vi "Main.vi"(10 "DAQ Type":enum16{"Hardware", "Simulation"}(ring), 11 "Module Admin":refnum<class "Delacor_lib_QMH_Module Admin.lvclass">) -> ()   [LabVIEW 2016, in "DAQ Hardware.lvlib"]
doc: "This template is based off of the Queued Message Handler design pattern and the Queued Message Handler project template that ships with LabVIEW.\n\nThe main difference is that the queue is private to this module and communication between modules is performed via Broadcast and Request events.\n\nRequest events are wrapped in public API methods and are handled in the Event Handling Loop (EHL) of this VI. Any module can register for Broadcast events sent by this module. The EHL generates messages based on user interface actions.\n\nThe Message Handling Loop (MHL) processes messages generated by the EHL, or by other messages. The messages are string values, so new messages can be added easily to the Message Cases case structure in the MHL. Each message cluster can also provide an optional value for Message Data, which is a variant that can be converted to whatever message-specific data is required.\n_____\nBased on DQMH Project Template 6.1.0.94."
uses:
  DAQ Hardware.lvlib
  <vilib>/Delacor/Delacor QMH/Libraries/Module Admin_class/Delacor_lib_QMH_Module Admin.lvclass
  Class/PXIe 6363/PXIe 6363.lvclass
  D:/common_ATE/Libraries/DAQ Hardware/Class/Abstract/Abstract.lvclass
  Module Data--cluster.ctl
  Class/Abstract/Abstract.lvclass
  User Interface/AI Channel Setting.ctl
  Timing AI DAQ Setting.ctl
  DI Channel Setting.ctl
  DO Channel Setting.ctl
  AO Channel Setting.ctl
  <vilib>/Delacor/Delacor QMH/Libraries/Message Queue_class/Delacor_lib_QMH_Message Queue.lvclass/Delacor_lib_QMH_Message Queue.ctl
  Stop Argument--cluster.ctl
  <vilib>/Delacor/Delacor QMH/Libraries/Module Admin_class/Delacor_lib_QMH_Module Admin.lvclass/Delacor_lib_QMH_Module Admin.ctl
  REQ Initialize AI Argument--cluster.ctl
  REQ Initialize AI (Reply Payload)--cluster.ctl
  REQ Initialize AO Argument--cluster.ctl
  REQ Initialize AO (Reply Payload)--cluster.ctl
  REQ Initialize DI Argument--cluster.ctl
  REQ Initialize DI (Reply Payload)--cluster.ctl
  REQ Initialize DO Argument--cluster.ctl
  REQ Initialize DO (Reply Payload)--cluster.ctl
  REQ Write DO Argument--cluster.ctl
  REQ Acquire AI Argument--cluster.ctl
  REQ Close Ref Argument--cluster.ctl
  REQ Write AO Argument--cluster.ctl
  REQ Update Sample Rate Argument--cluster.ctl
  REQ Acquire DI Argument--cluster.ctl
  <vilib>/Utility/miscctls.llb/LVPointTypeDef.ctl
  <vilib>/Delacor/Delacor QMH/Libraries/Message Queue_class/Delacor_lib_QMH_Enqueue Message (Single).vi
  <vilib>/Delacor/Delacor QMH/Libraries/Module Admin_class/Delacor_lib_QMH_Get External Launch.vi
  Support Global.vi
  <vilib>/Utility/error.llb/Error Cluster From Error Code.vi
  <vilib>/ErrorRing/Error Ring.xnode
  <vilib>/Delacor/Delacor QMH/Libraries/Message Queue_class/Delacor_lib_QMH_Message Queue.lvclass
  User Interface/User Interface.lvlib
panel:
  in  "Acquire DI":bool
  out "AI Data":dbl[][](graph)
  in  "Acquire AI":bool
  out "error out":errorcluster
  out "Status":string
  in  "Simulate MHL Error":bool
  in  "Simulate EHL Error":bool
  # "Other QMH Modules communicate with this Module via its Public API (wrappers for its Request Events).\n\nThis Module communicates with other Modules via its Broadcast Events.\nAny module that wants to get these messages, just registers for this module's Broadcast events."
  # "This template is for the Delacor Modified Queued Message Handler design pattern.\n\nSee the block diagram for more information on how to use this template."
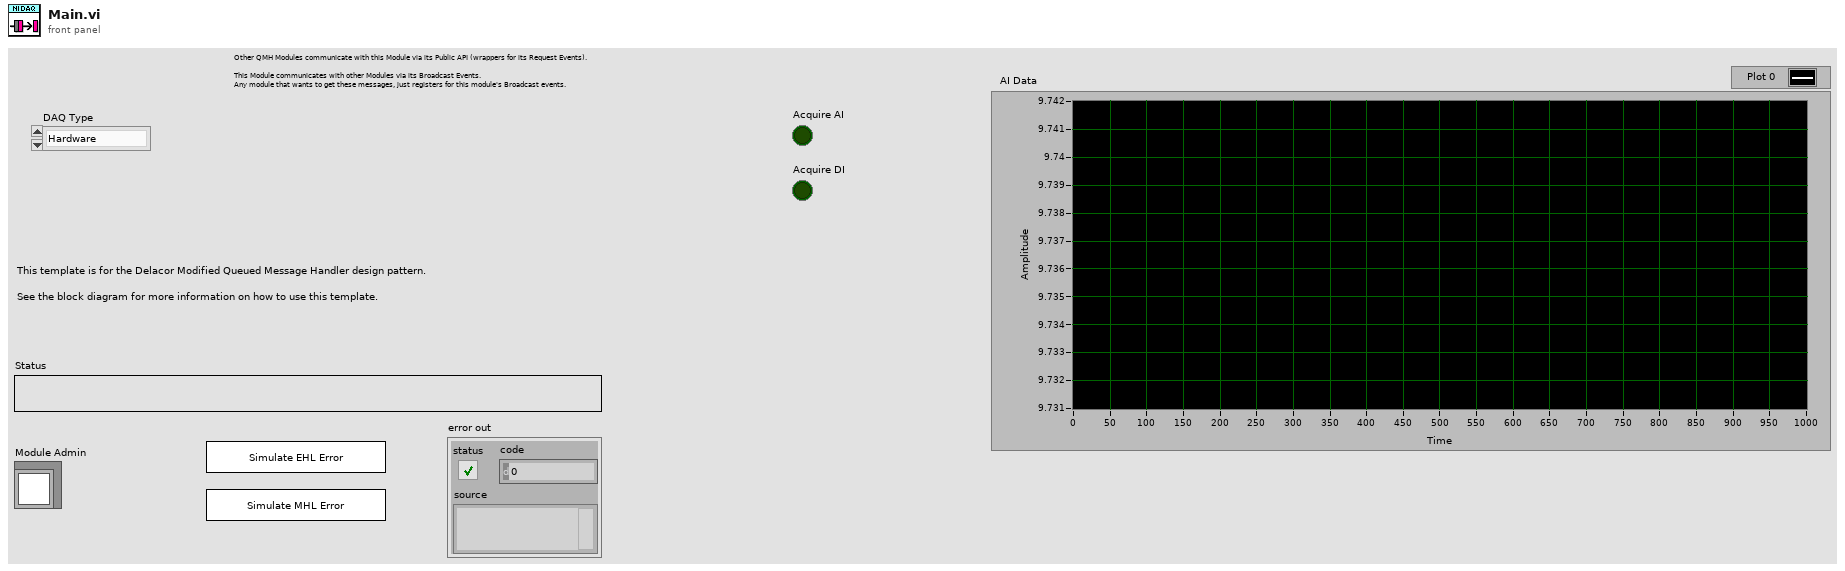
[diagram p1: front panel]
types:
  T1 = typedef "DAQ Hardware.lvlib/Module Data--cluster.ctl" = cluster{"Status":string, "Abstract.lvclass":refnum<class "Abstract.lvclass">, "AI Setting":T2, "Timing Parameter":T3, "DI Channel Setting":T4, "DO Channel Setting":T5, "AO Channel Setting":T6}
  T2 = typedef "DAQ Hardware.lvlib/AI Channel Setting.ctl" = cluster{"Physical Channel":string[], "Name to assign":string[], "input terminal configuration":enum16{"RSE", "NRSE", "Differential"}, "minimum value":dbl, "maximum value":dbl, "units":enum16{"Volts"}, "custom scale name":string, "sample mode":enum16{"Finite Samples", "Continuous Samples", "Hardware Timed Single Point"}, "rate":dbl, "samples per channel":dbl}
  T3 = typedef "DAQ Hardware.lvlib/Timing AI DAQ Setting.ctl" = cluster{"rate":dbl, "samples per channel":i32, "sample mode":i32}
  T4 = typedef "DAQ Hardware.lvlib/DI Channel Setting.ctl" = cluster{"DI Channel":string[]}
  T5 = typedef "DAQ Hardware.lvlib/DO Channel Setting.ctl" = cluster{"DO Channel":string[]}
  T6 = typedef "DAQ Hardware.lvlib/AO Channel Setting.ctl" = cluster{"AO Channel name":string[], "output terminal configuration":enum16{"RSE", "NRSE", "Differential"}, "minimum value":dbl, "maximum value":dbl, "units":enum16{"Volts"}, "name to assign":string[]}
  T7 = typedef "DAQ Hardware.lvlib/Request Events--cluster.ctl" = cluster{"Stop Module":refnum<user-event>, "Show Panel":refnum<user-event>, "Hide Panel":refnum<user-event>, "Get Module Execution Status":refnum<user-event>, "Show Diagram":refnum<user-event>, "REQ Initialize AI":refnum<user-event>, "REQ Initialize AO":refnum<user-event>, "REQ Initialize DI":refnum<user-event>, "REQ Initialize DO":refnum<user-event>, "REQ Write DO":refnum<user-event>, "REQ Acquire AI":refnum<user-event>, "REQ Close Ref":refnum<user-event>, "REQ Write AO":refnum<user-event>, "REQ Update Sample Rate":refnum<user-event>, "REQ Acquire DI":refnum<user-event>}
  T8 = enum32{"invalid lock state", "Not Locked", "Locked (No Password)", "Password-protected"}
  T9 = typedef "DAQ Hardware.lvlib/Stop Argument--cluster.ctl" = cluster{"Origin":string, "Exit via Stop Module Req?":bool, "Wait for Module to stop?":bool}
  T10 = typedef "DAQ Hardware.lvlib/REQ Initialize AI Argument--cluster.ctl" = cluster{"Wait Notifier":refnum<notifier>, "wait for reply":bool, "AI Setting":T2}
  T11 = typedef "DAQ Hardware.lvlib/REQ Initialize AO Argument--cluster.ctl" = cluster{"Boolean":bool, "Wait Notifier":refnum<notifier>, "wait for reply":bool, "AO Channel Setting":T6}
  T12 = typedef "DAQ Hardware.lvlib/REQ Initialize DI Argument--cluster.ctl" = cluster{"Boolean":bool, "Wait Notifier":refnum<notifier>, "wait for reply":bool, "DI Channel Setting":T4}
  T13 = typedef "DAQ Hardware.lvlib/REQ Initialize DO Argument--cluster.ctl" = cluster{"Boolean":bool, "Wait Notifier":refnum<notifier>, "wait for reply":bool, "DO Channel Setting":T5}
  T14 = typedef "DAQ Hardware.lvlib/REQ Write DO Argument--cluster.ctl" = cluster{"DO Value":bool[]}
  T15 = typedef "DAQ Hardware.lvlib/REQ Acquire AI Argument--cluster.ctl" = cluster{"Acquire AI":bool}
  T16 = typedef "DAQ Hardware.lvlib/REQ Close Ref Argument--cluster.ctl" = cluster{"Boolean":bool}
  T17 = typedef "DAQ Hardware.lvlib/REQ Write AO Argument--cluster.ctl" = cluster{"Value":dbl[]}
  T18 = typedef "DAQ Hardware.lvlib/REQ Update Sample Rate Argument--cluster.ctl" = cluster{"Timing Parameter":T3}
  T19 = typedef "DAQ Hardware.lvlib/REQ Acquire DI Argument--cluster.ctl" = cluster{"Acquire DI":bool}
  T20 = typedef "LVPointTypeDef.ctl" = cluster{"Horizontal":i16, "Vertical":i16}
  T21 = enum32{"Invalid", "Standard", "Closed", "Hidden", "Minimized", "Maximized"}
  T22 = typedef "DAQ Hardware.lvlib/REQ Initialize AI (Reply Payload)--cluster.ctl" = cluster{"error":errorcluster, "Connect?":bool}
  T23 = typedef "DAQ Hardware.lvlib/REQ Initialize AO (Reply Payload)--cluster.ctl" = cluster{"error":errorcluster, "Connect?":bool}
  T24 = typedef "DAQ Hardware.lvlib/REQ Initialize DI (Reply Payload)--cluster.ctl" = cluster{"error":errorcluster, "Connect?":bool}
  T25 = typedef "DAQ Hardware.lvlib/REQ Initialize DO (Reply Payload)--cluster.ctl" = cluster{"error":errorcluster, "Connect?":bool}
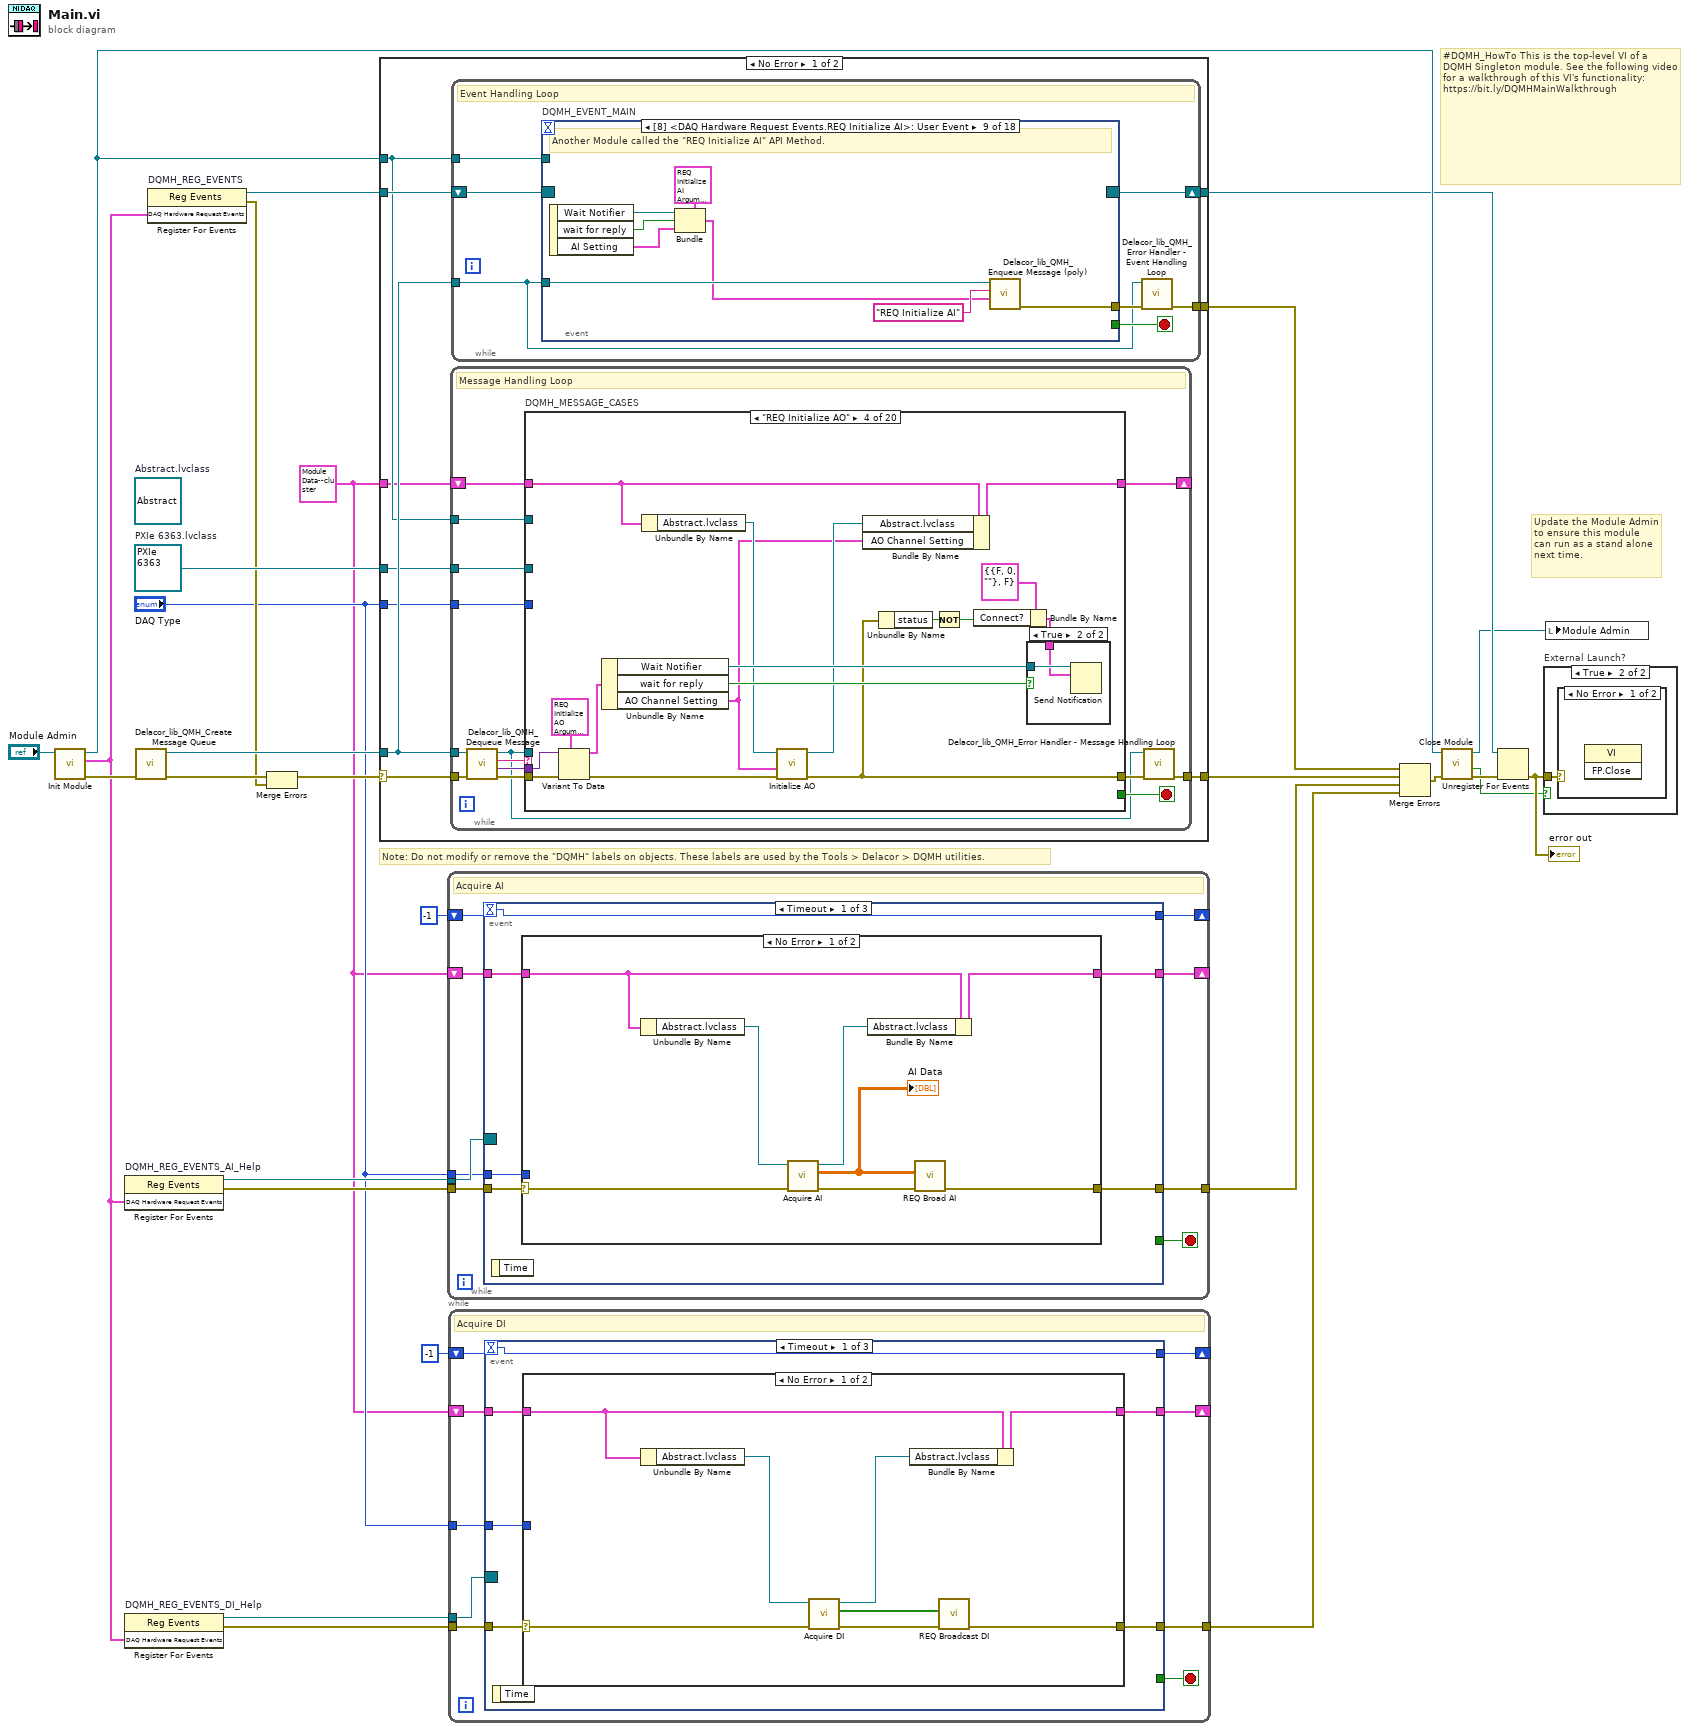
[diagram p0: block diagram]
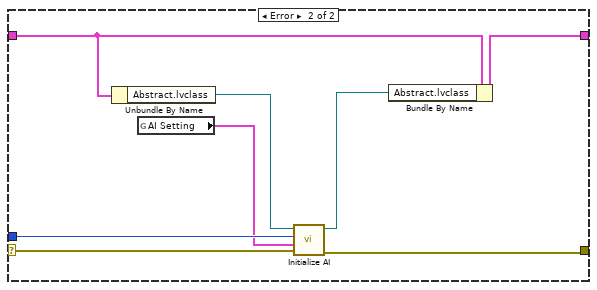
[diagram p2: hidden frame]
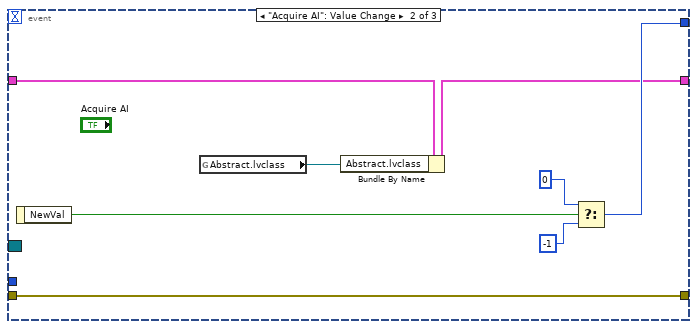
[diagram p3: hidden frame]
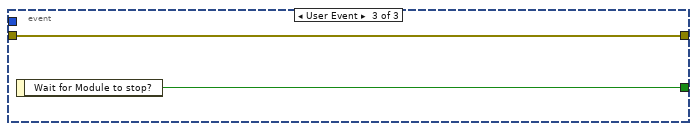
[diagram p4: hidden frame]
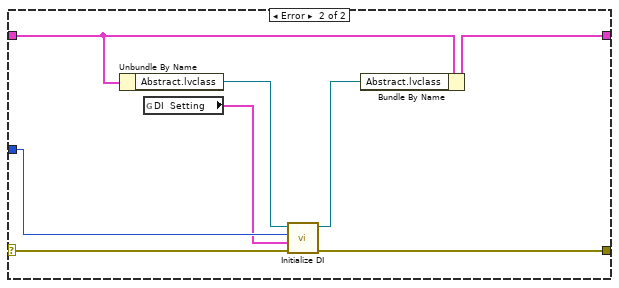
[diagram p5: hidden frame]
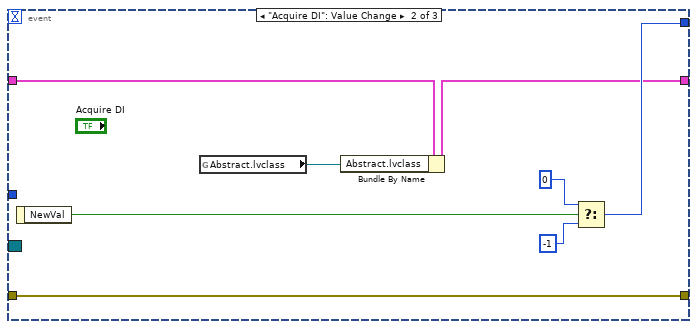
[diagram p6: hidden frame]
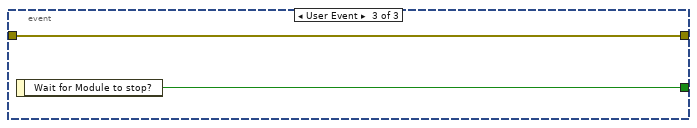
[diagram p7: hidden frame]
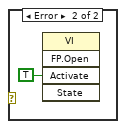
[diagram p9: hidden frame]
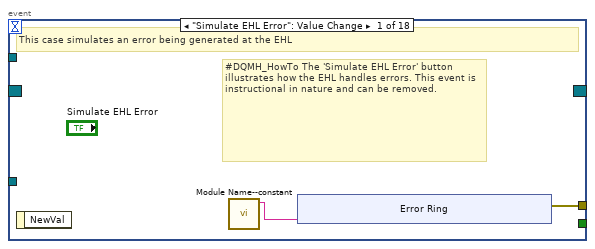
[diagram p10: hidden frame]
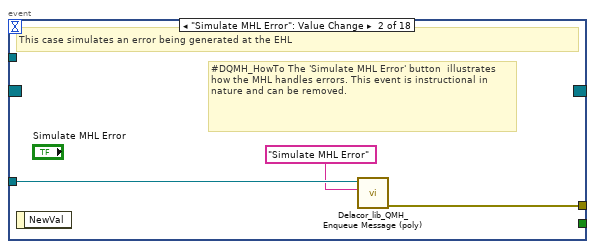
[diagram p11: hidden frame]
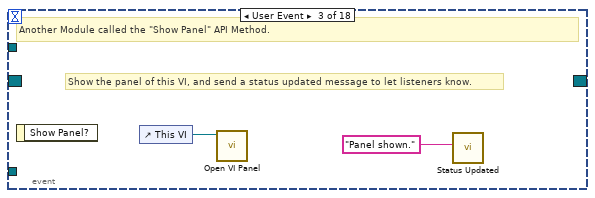
[diagram p12: hidden frame]
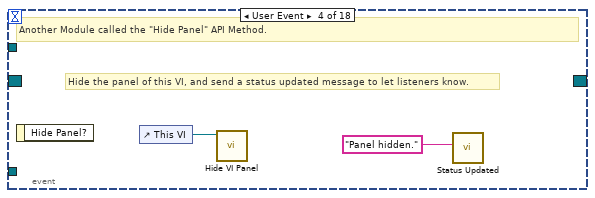
[diagram p13: hidden frame]
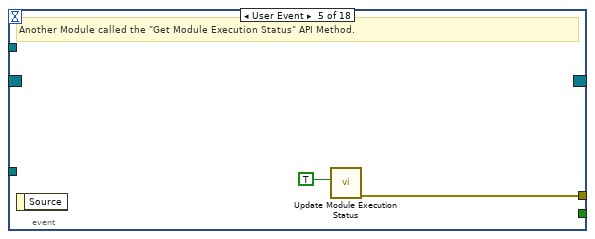
[diagram p14: hidden frame]
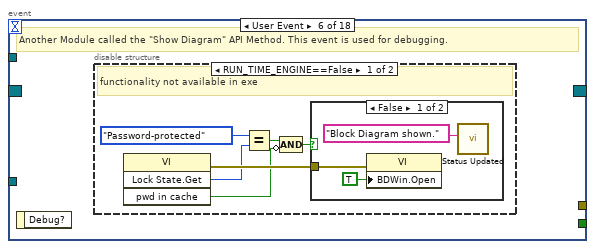
[diagram p15: hidden frame]
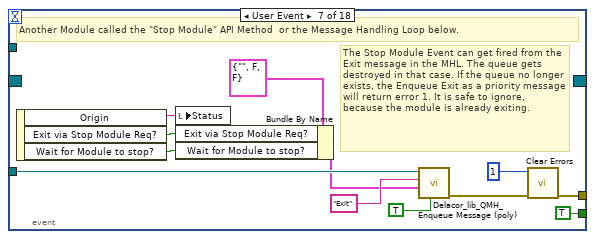
[diagram p18: hidden frame]
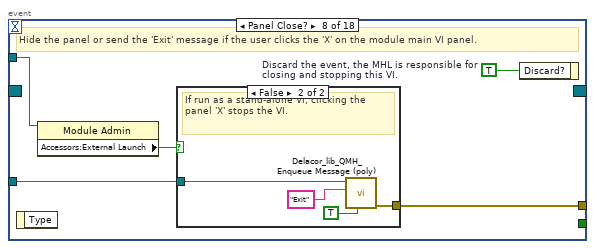
[diagram p19: hidden frame]
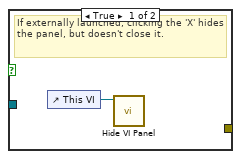
[diagram p20: hidden frame]
diagram:
  w1 = T1 {"Status"="", "Abstract.lvclass"=refnum, "AI Setting"={"Physical Channel"=["6363/ai0", "6363/ai1", "6363/ai2"], "Name to assign"=[], "input terminal configuration"=enum."RSE", "minimum value"=0.0, "maximum value"=10.0, "units"=enum."Volts", "custom scale name"="", "sample mode"=enum."Finite Samples", "rate"=5000.0, "samples per channel"=1000.0}, "Timing Parameter"={"rate"=1000.0, "samples per channel"=1000, "sample mode"=10123}, "DI Channel Setting"={"DI Channel"=[]}, "DO Channel Setting"={"DO Channel"=[]}, "AO Channel Setting"={"AO Channel name"=[], "output terminal configuration"=enum."RSE", "minimum value"=-10.0, "maximum value"=10.0, "units"=enum."Volts", "name to assign"=[]}} ("Data Cluster")
  w18 = refnum<class "PXIe 6363.lvclass"> refnum  # PXIe 6363.lvclass
  (unwired) refnum<class "Abstract.lvclass"> refnum  # Abstract.lvclass
  # "#DQMH_HowTo This is the top-level VI of a DQMH Singleton module. See the following video for a walkthrough of this VI's functionality: https://bit.ly/DQMHMainWalkthrough"
  # "Note: Do not modify or remove the \"DQMH\" labels on objects. These labels are used by the Tools > Delacor > DQMH utilities."
  # "Update the Module Admin to ensure this module can run as a stand alone next time."
  n1 = call "Init Module.vi"("Singleton Module Admin in"="Module Admin") -> ("error out"=w15:errorcluster, "DAQ Hardware Request Events"=w6:T7, "Singleton Module Admin out"=w23:refnum<class "Delacor_lib_QMH_Module Admin.lvclass">)  [unwired: 8 in]
  n2 = register-events "DQMH_REG_EVENTS_AI_Help"(w6) -> (reference out=w11:refnum<event-registration>, error out=w10:errorcluster)  [unwired: 2 in]
  n3 = register-events "DQMH_REG_EVENTS_DI_Help"(w6) -> (reference out=w5:refnum<event-registration>, error out=w4:errorcluster)  [unwired: 2 in]
  n4 = call <vilib>:"Delacor_lib_QMH_Create Message Queue.vi"("error in"=w15) -> ("error out"=w16:errorcluster, "Message Queue"=w17:refnum<class "Delacor_lib_QMH_Message Queue.lvclass">)  [unwired: 9 in]
  n5 = register-events "DQMH_REG_EVENTS"(w6) -> (reference out=w14:refnum<event-registration>, error out=w13:errorcluster)  [unwired: 2 in]
  n6 = Merge Errors(w16, w13) -> (w12:errorcluster)
  n7 = case shown="No Error" w12 {
    selector: w12 -> [w36 w453]
    tunnel: [w38 w452] -> w28
    tunnel: [w35 w458] -> w22
    tunnel: w14 -> [w34 w458]
    tunnel: w17 -> [w33 w451]
    tunnel: [w37 _] -> w26
    tunnel: w23 -> [w32 w454]
    tunnel: w18 -> [w31 _]
    tunnel: "DAQ Type" -> [w30 _]
    tunnel: w1 -> [w29 _]
    frame No Error {
      n8 = while {
        tunnel: w33 -> [w170]
        shift-right: [w174] -> _
        shift-left: w29 -> [w175]
        tunnel: w36 -> [w178]
        tunnel: [w176] -> w38
        tunnel: w32 -> [w168]
        tunnel: w31 -> [w167]
        tunnel: w30 -> [w166]
        stop <- w173 stop-if-true
        # "Message Handling Loop"
        n9 = call-dynamic "Delacor_lib_QMH_Dequeue Message.vi"("error in"=w178, "Message Queue in"=w170) -> ("error out"=w177:errorcluster, "Message Data"=w171:variant, "Message"=w172:string, "Message Queue out"=w169:refnum<class "Delacor_lib_QMH_Message Queue.lvclass">)  [unwired: 6 in]
        n10 = case "DQMH_MESSAGE_CASES" shown="\"REQ Initialize AO\"" w172 {
          selector: w172 -> [_ _ _ _ _ _ _ _ _ _ _ _ _ _ _ _ _ _ _ w438]
          tunnel: w169 -> [_ _ _ _ _ _ _ w291 _ w318 _ _ w372 w388 _ _ _ w408 w431 _]
          tunnel: w177 -> [w198 w202 w220 w239 w259 w279 w290 w303 w317 w330 w354 w371 w377 w387 w391 w393 w398 w415 w422 w440]
          tunnel: [w196 w202 w204 w226 w244 w266 w282 w292 w311 w319 w351 w358 w376 w386 w390 w393 w397 w411 w434 w441] -> w179
          tunnel: w175 -> [w187 w201 w207 w230 w250 w270 w286 w297 w310 w324 w350 w367 w379 w384 w389 w392 w395 w410 w430 w439]
          tunnel: [w186 w201 w211 w228 w248 w268 w286 w295 w310 w322 w348 w365 w379 w384 w389 w392 w395 w410 w430 w439] -> w174
          tunnel: [_ _ _ _ _ _ _ _ _ _ _ _ _ _ _ _ _ _ w429 _] -> w173
          tunnel: w171 -> [_ _ w219 w238 w258 w278 w289 w302 w316 w329 w353 w370 _ _ _ _ _ w409 w428 _]
          tunnel: w168 -> [w188 _ _ _ _ _ _ _ _ _ _ _ _ _ _ _ _ w407 w423 _]
          tunnel: w167 -> [w180 _ _ _ _ _ _ _ _ _ _ _ _ _ _ _ _ _ _ _]
          tunnel: w166 -> [_ _ w212 _ w243 w263 _ _ _ _ _ _ _ _ _ _ _ _ _ _]
          frame "Initialize" {
            w182 = "Initial Message" ("Initial Message")
            # "Initialize - Any operation that needs to be done before the module can receive messages. Synchronize Caller Events.vi will inform Start Module.vi that the module has launched and is ready to receive messages. Module Did Init.vi will broadcast that the module initialized."
            n11 = call "Synchronize Caller Events.vi"("error in (no error)"=w198, "Singleton Module Admin in"=w188) -> ("error out"=w197:errorcluster, "Singleton Module Admin out"=w183:refnum<class "Delacor_lib_QMH_Module Admin.lvclass">)  [unwired: 8 in]
            n12 = property class="Module Admin"(reference=w183) -> ("Accessors:External Launch"=w192:bool)  [unwired: 1 in, 2 out]
            n13 = Select(t=T21."Hidden" ("State"), s=w192, f=T21."Standard" ("State")) -> (s? t:f=w189:T21)
            n14 = call "Module Name--constant.vi"() -> ("Module Name"=w195:string)  [unwired: 11 in]
            n15 = property class="VI"("Front Panel.Title"=w195) -> (reference out=w194:refnum<vi>, error out=w200:errorcluster)  [unwired: 2 in]
            n16 = call "Module Name--constant.vi"() -> ("Module Name"=w184:string)  [unwired: 11 in]
            n17 = Bundle By Name(cluster=w187, "Status"=w182, "Abstract.lvclass"=w180) -> (w186:T1)
            n18 = invoke class="VI" method="FP.Open"(reference=w194, error in=w200, "State"=w189) -> (reference out=w193:refnum<vi>, error out=w199:errorcluster)  [unwired: 2 in, 3 out]
            n19 = call "Module Did Init.vi"("error in (no error)"=w197, "Initialized?"=TRUE, "Origin"=w184) -> ("error out"=w196:errorcluster)  [unwired: 8 in]
            n20 = invoke class="VI" method="FP.Center"(reference=w193, error in=w199) -> ()  [unwired: 1 in, 3 out]
            n21 = property on="Pane" class="Pane"("Origin"=T20 {"Horizontal"=0, "Vertical"=0}) -> ()  [unwired: 2 in, 2 out]
            "Status" <- w182
          }
          frame "---Module Specific---" {
            # "Separator -- The following cases handle messages specific to this Module."
          }
          frame "REQ Initialize AI" {
            n22 = Variant To Data(error in=w220, type=T10 {"Wait Notifier"=refnum, "wait for reply"=FALSE, "AI Setting"={"Physical Channel"=["6363/ai0", "6363/ai1", "6363/ai2"], "Name to assign"=[], "input terminal configuration"=enum."RSE", "minimum value"=0.0, "maximum value"=10.0, "units"=enum."Volts", "custom scale name"="", "sample mode"=enum."Finite Samples", "rate"=5000.0, "samples per channel"=1000.0}} ("REQ Initialize AI Argument"), Variant=w219) -> (data=w217:T10, error out=w203:errorcluster)
            n23 = Unbundle By Name(w217) -> ("Wait Notifier"=w216:refnum<notifier>, "wait for reply"=w215:bool, "AI Setting"=w205:T2)
            n24 = Unbundle By Name(w207) -> ("Abstract.lvclass"=w206:refnum<class "Abstract.lvclass">)
            n25 = call-dynamic "Initialize AI.vi"("error in (no error)"=w203, "AI Setting"=w205, "DAQ Type"=w212, "Abstract in"=w206) -> ("error out"=w204:errorcluster, "Abstract out"=w210:refnum<class "Abstract.lvclass">)  [unwired: 6 in]
            n26 = Unbundle By Name(w204) -> ("status"=w209:bool)
            n27 = global write "Support Global.vi" "AI Setting"(w205) -> ()
            n28 = Bundle By Name(cluster=w207, "Abstract.lvclass"=w210) -> (w211:T1)
            n29 = Not(x=w209) -> (.not. x?=w208:bool)
            n30 = Bundle By Name(cluster=T22 {"error"={"status"=FALSE, "code"=0, "source"=""}, "Connect?"=FALSE} ("REQ Initialize AI (Reply Payload)"), "Connect?"=w208) -> (w214:T22)
            n31 = case shown="True" w215 {
              tunnel: w216 -> [_ w222]
              tunnel: w214 -> [_ w221]
              frame False {
              }
              frame True {
                n32 = Send Notification(notification=w221, notifier=w222) -> ()  [unwired: 1 in, 2 out]
              }
            }
          }
          frame "REQ Initialize AO" {
            n33 = Variant To Data(error in=w239, type=T11 {"Boolean"=FALSE, "Wait Notifier"=refnum, "wait for reply"=FALSE, "AO Channel Setting"={"AO Channel name"=[], "output terminal configuration"=enum."RSE", "minimum value"=-10.0, "maximum value"=10.0, "units"=enum."Volts", "name to assign"=[]}} ("REQ Initialize AO Argument"), Variant=w238) -> (data=w236:T11, error out=w231:errorcluster)
            n34 = Unbundle By Name(w236) -> ("Wait Notifier"=w235:refnum<notifier>, "wait for reply"=w234:bool, "AO Channel Setting"=w223:T6)
            n35 = Unbundle By Name(w230) -> ("Abstract.lvclass"=w229:refnum<class "Abstract.lvclass">)
            n36 = call-dynamic "Initialize AO.vi"("error in (no error)"=w231, "AO Channel Setting"=w223, "Abstract in"=w229) -> ("error out"=w226:errorcluster, "Abstract out"=w227:refnum<class "Abstract.lvclass">)  [unwired: 7 in]
            n37 = Bundle By Name(cluster=w230, "Abstract.lvclass"=w227, "AO Channel Setting"=w223) -> (w228:T1)
            n38 = Unbundle By Name(w226) -> ("status"=w225:bool)
            n39 = Not(x=w225) -> (.not. x?=w224:bool)
            n40 = Bundle By Name(cluster=T23 {"error"={"status"=FALSE, "code"=0, "source"=""}, "Connect?"=FALSE} ("REQ Initialize AO (Reply Payload)"), "Connect?"=w224) -> (w233:T23)
            n41 = case shown="True" w234 {
              tunnel: w235 -> [_ w241]
              tunnel: w233 -> [_ w240]
              frame False {
              }
              frame True {
                n42 = Send Notification(notification=w240, notifier=w241) -> ()  [unwired: 1 in, 2 out]
              }
            }
          }
          frame "REQ Initialize DI" {
            n43 = Variant To Data(error in=w259, type=T12 {"Boolean"=FALSE, "Wait Notifier"=refnum, "wait for reply"=FALSE, "DI Channel Setting"={"DI Channel"=[]}} ("REQ Initialize DI Argument"), Variant=w258) -> (data=w256:T12, error out=w251:errorcluster)
            n44 = Unbundle By Name(w250) -> ("Abstract.lvclass"=w249:refnum<class "Abstract.lvclass">)
            n45 = Unbundle By Name(w256) -> ("Wait Notifier"=w255:refnum<notifier>, "wait for reply"=w254:bool, "DI Channel Setting"=w242:T4)
            n46 = call-dynamic "Initialize DI.vi"("error in (no error)"=w251, "DI Channel Setting"=w242, "DAQ Type"=w243, "Abstract in"=w249) -> ("error out"=w244:errorcluster, "Abstract out"=w247:refnum<class "Abstract.lvclass">)  [unwired: 6 in]
            n47 = Unbundle By Name(w244) -> ("status"=w246:bool)
            n48 = global write "Support Global.vi" "DI  Setting"(w242) -> ()
            n49 = Bundle By Name(cluster=w250, "Abstract.lvclass"=w247) -> (w248:T1)
            n50 = Not(x=w246) -> (.not. x?=w245:bool)
            n51 = Bundle By Name(cluster=T24 {"error"={"status"=FALSE, "code"=0, "source"=""}, "Connect?"=FALSE} ("REQ Initialize DI (Reply Payload)"), "Connect?"=w245) -> (w253:T24)
            n52 = case shown="True" w254 {
              tunnel: w255 -> [_ w261]
              tunnel: w253 -> [_ w260]
              frame False {
              }
              frame True {
                n53 = Send Notification(notification=w260, notifier=w261) -> ()  [unwired: 1 in, 2 out]
              }
            }
          }
          frame "REQ Initialize DO" {
            n54 = Variant To Data(error in=w279, type=T13 {"Boolean"=FALSE, "Wait Notifier"=refnum, "wait for reply"=FALSE, "DO Channel Setting"={"DO Channel"=[]}} ("REQ Initialize DO Argument"), Variant=w278) -> (data=w276:T13, error out=w271:errorcluster)
            n55 = Unbundle By Name(w276) -> ("Wait Notifier"=w275:refnum<notifier>, "wait for reply"=w274:bool, "DO Channel Setting"=w262:T5)
            n56 = Unbundle By Name(w270) -> ("Abstract.lvclass"=w269:refnum<class "Abstract.lvclass">)
            n57 = call-dynamic "Initialize DO.vi"("error in (no error)"=w271, "DO Channel Setting"=w262, "DAQ Type"=w263, "Abstract in"=w269) -> ("error out"=w266:errorcluster, "Abstract out"=w267:refnum<class "Abstract.lvclass">)  [unwired: 6 in]
            n58 = Unbundle By Name(w266) -> ("status"=w265:bool)
            n59 = Bundle By Name(cluster=w270, "Abstract.lvclass"=w267, "DO Channel Setting"=w262) -> (w268:T1)
            n60 = Not(x=w265) -> (.not. x?=w264:bool)
            n61 = Bundle By Name(cluster=T25 {"error"={"status"=FALSE, "code"=0, "source"=""}, "Connect?"=FALSE} ("REQ Initialize DO (Reply Payload)"), "Connect?"=w264) -> (w273:T25)
            n62 = case shown="True" w274 {
              tunnel: w275 -> [_ w281]
              tunnel: w273 -> [_ w280]
              frame False {
              }
              frame True {
                n63 = Send Notification(notification=w280, notifier=w281) -> ()  [unwired: 1 in, 2 out]
              }
            }
          }
          frame "REQ Acquire AI" {
            n64 = Variant To Data(error in=w290, type=T15 {"Acquire AI"=FALSE} ("REQ Acquire AI Argument"), Variant=w289) -> (data=w287:T15, error out=w283:errorcluster)
            n65 = Unbundle By Name(w287) -> ("Acquire AI"=w284:bool)
            n66 = Unbundle By Name(w286) -> ("Abstract.lvclass"=w285:refnum<class "Abstract.lvclass">)
            n67 = global write "Support Global.vi" "Abstract.lvclass"(w285) -> ()
            n68 = property on="Acquire AI" class="Bool (strict)"(error in=w283, "Val(Sgnl)"=w284) -> (error out=w282:errorcluster)  [unwired: 1 in, 1 out]
          }
          frame "REQ Write AO" {
            n69 = Variant To Data(error in=w303, type=T17 {"Value"=[]} ("REQ Write AO Argument"), Variant=w302) -> (data=w300:T17, error out=w299:errorcluster)
            n70 = Unbundle By Name(w300) -> ("Value"=w298:dbl[])
            n71 = Unbundle By Name(w297) -> ("Abstract.lvclass"=w296:refnum<class "Abstract.lvclass">)
            n72 = call-dynamic "Write AO Value.vi"("error in (no error)"=w299, "Value"=w298, "Abstract in"=w296) -> ("error out"=w293:errorcluster, "Abstract out"=w294:refnum<class "Abstract.lvclass">)  [unwired: 7 in]
            n73 = Bundle By Name(cluster=w297, "Abstract.lvclass"=w294) -> (w295:T1)
            n74 = case shown="Error" w293 {
              selector: w293 -> [w304 w307]
              tunnel: [w304 w306] -> w292
              tunnel: w291 -> [_ w305]
              frame No Error {
              }
              frame Error {
                n75 = call-poly <vilib>:"Delacor_lib_QMH_Enqueue Message (poly).vi"("error in"=w307, "Message"="REQ Reconnect AO", "Message Queue in"=w305) -> ("error out"=w306:errorcluster)  [unwired: 7 in, 1 out]
              }
            }
          }
          frame "REQ Acquire DI" {
            n76 = Variant To Data(error in=w317, type=T19 {"Acquire DI"=FALSE} ("REQ Acquire DI Argument"), Variant=w316) -> (data=w314:T19, error out=w313:errorcluster)
            n77 = Unbundle By Name(w314) -> ("Acquire DI"=w312:bool)
            n78 = Unbundle By Name(w310) -> ("Abstract.lvclass"=w309:refnum<class "Abstract.lvclass">)
            n79 = global write "Support Global.vi" "Abstract.lvclass"(w309) -> ()
            n80 = property on="Acquire DI" class="Bool (strict)"(error in=w313, "Val(Sgnl)"=w312) -> (error out=w311:errorcluster)  [unwired: 1 in, 1 out]
          }
          frame "REQ Write DO" {
            n81 = Variant To Data(error in=w330, type=T14 {"DO Value"=[]} ("REQ Write DO Argument"), Variant=w329) -> (data=w327:T14, error out=w326:errorcluster)
            n82 = Unbundle By Name(w327) -> ("DO Value"=w325:bool[])
            n83 = Unbundle By Name(w324) -> ("Abstract.lvclass"=w323:refnum<class "Abstract.lvclass">)
            n84 = call-dynamic "Write DO Value.vi"("error in (no error)"=w326, "DO Value"=w325, "Abstract in"=w323) -> ("error out"=w320:errorcluster, "Abstract out"=w321:refnum<class "Abstract.lvclass">)  [unwired: 7 in]
            n85 = Bundle By Name(cluster=w324, "Abstract.lvclass"=w321) -> (w322:T1)
            n86 = case shown="Error" w320 {
              selector: w320 -> [w331 w334]
              tunnel: [w331 w333] -> w319
              tunnel: w318 -> [_ w332]
              frame No Error {
              }
              frame Error {
                n87 = call-poly <vilib>:"Delacor_lib_QMH_Enqueue Message (poly).vi"("error in"=w334, "Message"="REQ Initialize DO", "Message Queue in"=w332) -> ("error out"=w333:errorcluster)  [unwired: 7 in, 1 out]
              }
            }
          }
          frame "REQ Close Ref" {
            n88 = Variant To Data(error in=w354, type=T16 {"Boolean"=FALSE} ("REQ Close Ref Argument"), Variant=w353) -> (error out=w340:errorcluster)  [unwired: 1 out]
            n89 = property on="Acquire AI" class="Bool (strict)"(error in=w340, "Val(Sgnl)"=FALSE ("Value (Signaling)")) -> (error out=w339:errorcluster)  [unwired: 1 in, 1 out]
            n90 = Unbundle By Name(w350) -> ("Abstract.lvclass"=w349:refnum<class "Abstract.lvclass">)
            n91 = property on="Acquire DI" class="Bool (strict)"(error in=w339, "Val(Sgnl)"=FALSE ("Value (Signaling)")) -> (error out=w338:errorcluster)  [unwired: 1 in, 1 out]
            n92 = call-dynamic "Close AO.vi"("error in (no error)"=w338, "Abstract in"=w349) -> ("error out"=w346:errorcluster, "Abstract out"=w343:refnum<class "Abstract.lvclass">)  [unwired: 8 in]
            n93 = call-dynamic "Close DI.vi"("error in (no error)"=w346, "Abstract in"=w343) -> ("error out"=w345:errorcluster, "Abstract out"=w342:refnum<class "Abstract.lvclass">)  [unwired: 8 in]
            n94 = call-dynamic "Close DO.vi"("error in (no error)"=w345, "Abstract in"=w342) -> ("error out"=w344:errorcluster, "Abstract out"=w341:refnum<class "Abstract.lvclass">)  [unwired: 8 in]
            n95 = call-dynamic "Close AI.vi"("error in (no error)"=w344, "Abstract in"=w341) -> ("error out"=w351:errorcluster, "Abstract out"=w347:refnum<class "Abstract.lvclass">)  [unwired: 8 in]
            n96 = Bundle By Name(cluster=w350, "Abstract.lvclass"=w347) -> (w348:T1)
          }
          frame "REQ Update Sample Rate" {
            n97 = Variant To Data(error in=w371, type=T18 {"Timing Parameter"={"rate"=1000.0, "samples per channel"=1000, "sample mode"=10123}} ("REQ Update Sample Rate Argument"), Variant=w370) -> (data=w368:T18, error out=w362:errorcluster)
            n98 = Unbundle By Name(w368) -> ("Timing Parameter"=w364:T3)
            n99 = Unbundle By Name(w367) -> ("Abstract.lvclass"=w366:refnum<class "Abstract.lvclass">)
            n100 = property on="Acquire AI" class="Bool (strict)"(error in=w362, "Val(Sgnl)"=FALSE ("Value (Signaling)")) -> (error out=w360:errorcluster)  [unwired: 1 in, 1 out]
            n101 = call-dynamic "Update Sampling Rate.vi"("error in (no error)"=w360, "Timing Parameter"=w364, "Abstract in"=w366) -> ("error out"=w357:errorcluster, "Abstract out"=w363:refnum<class "Abstract.lvclass">)  [unwired: 7 in]
            n102 = call "Stall Data Flow.vi"("milliseconds to wait"=u32 100, "error in (no error)"=w357) -> ("error out"=w356:errorcluster)  [unwired: 9 in]
            n103 = global write "Support Global.vi" "Abstract.lvclass"(w363) -> ()
            n104 = Bundle By Name(cluster=w367, "Abstract.lvclass"=w363) -> (w365:T1)
            n105 = property on="Acquire AI" class="Bool (strict)"(error in=w356, "Val(Sgnl)"=TRUE ("Value (Signaling)")) -> (error out=w358:errorcluster)  [unwired: 1 in, 1 out]
          }
          frame "REQ Reconnect DO" {
            # "Duplicate this frame when creating new messages.  Change this comment in the duplicated frame to describe this message."
            n106 = Unbundle By Name(w379) -> ("DO Channel Setting"=w374:T5)
            n107 = Bundle By Name(cluster=T13 {"Boolean"=FALSE, "Wait Notifier"=refnum, "wait for reply"=FALSE, "DO Channel Setting"={"DO Channel"=[]}} ("REQ Initialize DO Argument"), "DO Channel Setting"=w374) -> (w373:T13)
            n108 = call-poly <vilib>:"Delacor_lib_QMH_Enqueue Message (poly).vi"("error in"=w377, "Message Data"=w373, "Message"="REQ Initialize DO", "Message Queue in"=w372) -> ("error out"=w376:errorcluster)  [unwired: 6 in, 1 out]
          }
          frame "REQ Reconnect AO" {
            # "Duplicate this frame when creating new messages.  Change this comment in the duplicated frame to describe this message."
            n109 = Unbundle By Name(w384) -> ("AO Channel Setting"=w382:T6)
            n110 = Bundle By Name(cluster=T11 {"Boolean"=FALSE, "Wait Notifier"=refnum, "wait for reply"=FALSE, "AO Channel Setting"={"AO Channel name"=[], "output terminal configuration"=enum."RSE", "minimum value"=-10.0, "maximum value"=10.0, "units"=enum."Volts", "name to assign"=[]}} ("REQ Initialize AO Argument"), "AO Channel Setting"=w382) -> (w381:T11)
            n111 = call-poly <vilib>:"Delacor_lib_QMH_Enqueue Message (poly).vi"("error in"=w387, "Message Data"=w381, "Message"="REQ Initialize AO", "Message Queue in"=w388) -> ("error out"=w386:errorcluster)  [unwired: 6 in, 1 out]
            n112 = Wait (ms)(milliseconds to wait=u32 1000) -> ()  [unwired: 1 out]
          }
          frame "---Copy This Frame---" {
            # "Duplicate this frame when creating new messages.  Change this comment in the duplicated frame to describe this message."
            n113 = Merge Errors(w391) -> (w390:errorcluster)
          }
          frame "---Exit and Error Handling---" {
            # "Separator - The following cases handle errors and exit messages."
          }
          frame "Simulate MHL Error" {
            # "#DQMH_HowTo The 'Simulate MHL Error' button  illustrates how the MHL handles errors. This event is instructional in nature and can be removed."
            # "Simulate an error occurring at the MHL"
            n114 = call "Module Name--constant.vi"() -> ("Module Name"=w394:string)  [unwired: 11 in]
            n115 = xnode "Error Ring"("parameter 0"=w394) -> ("error out"=w396:errorcluster)
            n116 = Merge Errors(w398, w396) -> (w397:errorcluster)
          }
          frame "Error" {
            (unwired) "REQ Reconnect "
            # "Error - Check the error message data and respond accordingly. This message is sent by the \"Error Handler\" VIs at the end of each loop in this application."
            n117 = property class="Module Admin"(reference=w407) -> ("Accessors:External Launch"=w406:bool)  [unwired: 1 in, 2 out]
            n118 = Variant To Data(error in=w415, type=errorcluster {"status"=FALSE, "code"=0, "source"=""} ("error constant"), Variant=w409) -> (data=w416:errorcluster, error out=w413:errorcluster)
            n119 = call "Error Reported.vi"("Error"=w416) -> ()  [unwired: 10 in, 1 out]
            n120 = case shown="False" w406 {
              tunnel: [w421 _] -> w412
              tunnel: w408 -> [w419 _]
              tunnel: w416 -> [w420 _]
              frame False {
                n121 = call <vilib>:"Simple Error Handler.vi"("error in (no error)"=w420) -> ()  [unwired: 4 in, 5 out]
                n122 = call-poly <vilib>:"Delacor_lib_QMH_Enqueue Message (poly).vi"("Priority Message? (F)"=TRUE, "Message"="Exit", "Message Queue in"=w419) -> ("error out"=w421:errorcluster)  [unwired: 7 in, 1 out]
              }
              frame True {
                # "If the module was launched externally, calling the Error Reported broadcast VI is the only action performed by the \"Error\" message. The module's caller can then process the error appropriately."
              }
            }
            n123 = Merge Errors(w413, w412) -> (w411:errorcluster)
            n124 = local write "error out"(w411) -> ()
          }
          frame "Exit" {
            w427 = 91  # 91: not all Exit messages will have an argument
            w429 = TRUE  # Stop the VI
            # "Release the message queue reference"
            # "#CodeNeeded - Add any required cleanup code here"
            # "Exit - Exit the application."
            n125 = Variant To Data(error in=w422, type=T9 {"Origin"="", "Exit via Stop Module Req?"=FALSE, "Wait for Module to stop?"=FALSE} ("Stop Argument"), Variant=w428) -> (data=w425:T9, error out=w433:errorcluster)
            n126 = call <vilib>:"Clear Errors.vi"("error in (no error)"=w433, "specific error code to clear (0: all)"=w427) -> ("error out"=w436:errorcluster)  [unwired: 4 in, 1 out]
            n127 = control-ref of="This VI"() -> (w424:refnum<vi>)
            n128 = call-dynamic "Delacor_lib_QMH_Release Message Queue.vi"("error in"=w436, "Message Queue"=w431) -> ("error out"=w435:errorcluster)  [unwired: 9 in]
            n129 = call "Handle Exit.vi"("Stop Argument"=w425, "Admin in"=w423, "VI reference"=w424) -> ("error out"=w432:errorcluster)  [unwired: 7 in, 1 out]
            n130 = Merge Errors(w435, w432) -> (w434:errorcluster)
          }
          frame Default {
            # "'Default' case only runs if there is a message that isn't defined in any of the other cases.  Output a programming error."
            n131 = call "Module Name--constant.vi"() -> ("Module Name"=w437:string)  [unwired: 11 in]
            n132 = xnode "Error Ring"("parameter 0"=w438, "parameter 1"=w437) -> ("error out"=w442:errorcluster)
            n133 = Merge Errors(w440, w442) -> (w441:errorcluster)
          }
        }
        n134 = call-dynamic "Delacor_lib_QMH_Error Handler - Message Handling Loop.vi"("error in"=w179, "Message Queue in"=w169) -> ("dup error in"=w176:errorcluster)  [unwired: 8 in, 1 out]
      }
      n135 = while {
        tunnel: w33 -> [w39]
        shift-right: [w42] -> w35
        shift-left: w34 -> [w43]
        tunnel: [w44] -> w37
        tunnel: w32 -> [w40]
        stop <- w41 stop-if-true
        # "Event Handling Loop"
        n136 = event "DQMH_EVENT_MAIN" shown="[8] <DAQ Hardware Request Events.REQ Initialize AI>: User Event" {
          selector: w43 -> [_ _ _ _ _ _ _ _ _ _ _ _ _ _ _ _ _ _]
          dyn-events: [_ _ _ _ _ _ _ _ _ _ _ _ _ _ _ _ _ _] -> w42
          timeout: _ -> [_ _ _ _ _ _ _ _ _ _ _ _ _ _ _ _ _ _]
          tunnel: [_ _ _ _ _ _ TRUE ("Discard?") _ _ _ _ _ _ _ _ _ _ _] -> w41
          tunnel: w39 -> [_ w56 _ _ _ _ w80 w87 w102 w111 w120 w129 w135 w141 w147 w153 w159 w165]
          tunnel: [w47 w57 _ _ w63 _ w83 w89 w98 w106 w115 w124 w130 w136 w142 w149 w154 w160] -> w45
          tunnel: w40 -> [_ _ _ _ _ _ _ w86 _ _ _ _ _ _ _ _ _ _]
          event "Simulate EHL Error": Value Change {
            # "#DQMH_HowTo The 'Simulate EHL Error' button  illustrates how the EHL handles errors. This event is instructional in nature and can be removed."
            # "This case simulates an error being generated at the EHL"
            n137 = event-data() -> ()  [unwired: 1 in, 1 out]
            n138 = call "Module Name--constant.vi"() -> ("Module Name"=w46:string)  [unwired: 11 in]
            n139 = xnode "Error Ring"("parameter 0"=w46) -> ("error out"=w47:errorcluster)
          }
          event "Simulate MHL Error": Value Change {
            # "#DQMH_HowTo The 'Simulate MHL Error' button  illustrates how the MHL handles errors. This event is instructional in nature and can be removed."
            # "This case simulates an error being generated at the EHL"
            n140 = event-data() -> ()  [unwired: 1 in, 1 out]
            n141 = call-poly <vilib>:"Delacor_lib_QMH_Enqueue Message (poly).vi"("Message"="Simulate MHL Error", "Message Queue in"=w56) -> ("error out"=w57:errorcluster)  [unwired: 8 in, 1 out]
          }
          event User Event {
            # "Show the panel of this VI, and send a status updated message to let listeners know."
            # "Another Module called the \"Show Panel\" API Method."
            n142 = event-data() -> ()  [unwired: 1 in, 1 out]
            n143 = control-ref of="This VI"() -> (w59:refnum<vi>)
            n144 = call "Open VI Panel.vi"("VI"=w59) -> ()  [unwired: 10 in, 1 out]
            n145 = call "Status Updated.vi"("Status"="Panel shown." ("format string")) -> ()  [unwired: 10 in, 1 out]
          }
          event User Event {
            # "Hide the panel of this VI, and send a status updated message to let listeners know."
            # "Another Module called the \"Hide Panel\" API Method."
            n146 = event-data() -> ()  [unwired: 1 in, 1 out]
            n147 = control-ref of="This VI"() -> (w61:refnum<vi>)
            n148 = call "Hide VI Panel.vi"("VI"=w61) -> ()  [unwired: 10 in, 1 out]
            n149 = call "Status Updated.vi"("Status"="Panel hidden." ("format string")) -> ()  [unwired: 10 in, 1 out]
          }
          event User Event {
            # "Another Module called the \"Get Module Execution Status\" API Method."
            n150 = event-data() -> ()  [unwired: 1 in, 1 out]
            n151 = call "Update Module Execution Status.vi"("Running?"=TRUE) -> ("error out"=w63:errorcluster)  [unwired: 10 in]
          }
          event User Event {
            # "Another Module called the \"Show Diagram\" API Method. This event is used for debugging."
            n152 = event-data() -> ()  [unwired: 1 in, 1 out]
            n153 = disable-structure shown="RUN_TIME_ENGINE==False" {
              frame condition #0 (active) {
                # "functionality not available in exe"
                n154 = invoke class="VI" method="Lock State.Get"() -> (error out=w69:errorcluster, "Get Lock State"=w68:T8, "pwd in cache"=w65:bool)  [unwired: 4 in, 1 out]
                n155 = Equal?(x=T8."Password-protected", y=w68) -> (x = y?=w66:bool)
                n156 = Compound Arithmetic op=AND(w66, invert w65) -> (w64:bool)
                n157 = case shown="False" w64 {
                  tunnel: w69 -> [w72 _]
                  frame False {
                    n158 = property class="VI"(error in=w72, "BDWin.Open"=TRUE ("Block Diagram Window:Open")) -> ()  [unwired: 1 in, 2 out]
                    n159 = call "Status Updated.vi"("Status"="Block Diagram shown." ("format string")) -> ()  [unwired: 10 in, 1 out]
                  }
                  frame True {
                    # "Password-protected VI, and the password is not in the cache. Do not show the diagram."
                  }
                }
              }
              frame condition #1 {
              }
            }
          }
          event User Event {
            # "The Stop Module Event can get fired from the Exit message in the MHL. The queue gets destroyed in that case. If the queue no longer exists, the Enqueue Exit as a priority message will return error 1. It is safe to ignore, because the module is already exiting."
            # "Another Module called the \"Stop Module\" API Method  or the Message Handling Loop below."
            n160 = event-data() -> ("Origin"=w79:string, "Exit via Stop Module Req?"=w75:bool, "Wait for Module to stop?"=w74:bool)  [unwired: 1 in]
            n161 = local write "Status"(w79) -> ()
            n162 = Bundle By Name(cluster=T9 {"Origin"="", "Exit via Stop Module Req?"=FALSE, "Wait for Module to stop?"=FALSE} ("Stop Argument"), "Exit via Stop Module Req?"=w75, "Wait for Module to stop?"=w74) -> (w73:T9)
            n163 = call-poly <vilib>:"Delacor_lib_QMH_Enqueue Message (poly).vi"("Priority Message? (F)"=TRUE, "Message Data"=w73, "Message"="Exit", "Message Queue in"=w80) -> ("error out"=w84:errorcluster)  [unwired: 6 in, 1 out]
            n164 = call <vilib>:"Clear Errors.vi"("error in (no error)"=w84, "specific error code to clear (0: all)"=1) -> ("error out"=w83:errorcluster)  [unwired: 4 in, 1 out]
          }
          event Panel Close? {
            w88 = TRUE  # Discard the event, the MHL is responsible for closing and stopping this VI.
            # "Hide the panel or send the 'Exit' message if the user clicks the 'X' on the module main VI panel."
            n165 = event-data() -> ()  [unwired: 1 in, 1 out]
            n166 = property class="Module Admin"(reference=w86) -> ("Accessors:External Launch"=w85:bool)  [unwired: 1 in, 2 out]
            n167 = case shown="False" w85 {
              tunnel: w87 -> [_ w93]
              tunnel: [_ w94] -> w89
              frame True {
                # "If externally launched, clicking the 'X' hides the panel, but doesn't close it."
                n168 = control-ref of="This VI"() -> (w90:refnum<vi>)
                n169 = call "Hide VI Panel.vi"("VI"=w90) -> ()  [unwired: 10 in, 1 out]
              }
              frame False {
                # "If run as a stand-alone VI, clicking the panel 'X' stops the VI."
                n170 = call-poly <vilib>:"Delacor_lib_QMH_Enqueue Message (poly).vi"("Priority Message? (F)"=TRUE, "Message"="Exit", "Message Queue in"=w93) -> ("error out"=w94:errorcluster)  [unwired: 7 in, 1 out]
              }
            }
            n171 = event-data("Discard?"=w88) -> ()  [unwired: 1 in, 1 out]
          }
          event User Event {
            # "Another Module called the \"REQ Initialize AI\" API Method."
            n172 = event-data() -> ("Wait Notifier"=w97:refnum<notifier>, "wait for reply"=w96:bool, "AI Setting"=w95:T2)  [unwired: 1 in]
            n173 = Bundle(cluster=T10 {"Wait Notifier"=refnum, "wait for reply"=FALSE, "AI Setting"={"Physical Channel"=["6363/ai0", "6363/ai1", "6363/ai2"], "Name to assign"=[], "input terminal configuration"=enum."RSE", "minimum value"=0.0, "maximum value"=10.0, "units"=enum."Volts", "custom scale name"="", "sample mode"=enum."Finite Samples", "rate"=5000.0, "samples per channel"=1000.0}} ("REQ Initialize AI Argument"), "Wait Notifier"=w97, "wait for reply"=w96, "AI Setting"=w95) -> (w99:T10)
            n174 = call-poly <vilib>:"Delacor_lib_QMH_Enqueue Message (poly).vi"("Message Data"=w99, "Message"="REQ Initialize AI", "Message Queue in"=w102) -> ("error out"=w98:errorcluster)  [unwired: 7 in, 1 out]
          }
          event User Event {
            # "Another Module called the \"REQ Initialize AO\" API Method."
            n175 = event-data() -> ("Boolean"=w107:bool, "Wait Notifier"=w105:refnum<notifier>, "wait for reply"=w104:bool, "AO Channel Setting"=w103:T6)  [unwired: 1 in]
            n176 = Bundle(cluster=T11 {"Boolean"=FALSE, "Wait Notifier"=refnum, "wait for reply"=FALSE, "AO Channel Setting"={"AO Channel name"=[], "output terminal configuration"=enum."RSE", "minimum value"=-10.0, "maximum value"=10.0, "units"=enum."Volts", "name to assign"=[]}} ("REQ Initialize AO Argument"), "Boolean"=w107, "Wait Notifier"=w105, "wait for reply"=w104, "AO Channel Setting"=w103) -> (w108:T11)
            n177 = call-poly <vilib>:"Delacor_lib_QMH_Enqueue Message (poly).vi"("Message Data"=w108, "Message"="REQ Initialize AO", "Message Queue in"=w111) -> ("error out"=w106:errorcluster)  [unwired: 7 in, 1 out]
          }
          event User Event {
            # "Another Module called the \"REQ Initialize DI\" API Method."
            n178 = event-data() -> ("Boolean"=w116:bool, "Wait Notifier"=w114:refnum<notifier>, "wait for reply"=w113:bool, "DI Channel Setting"=w112:T4)  [unwired: 1 in]
            n179 = Bundle(cluster=T12 {"Boolean"=FALSE, "Wait Notifier"=refnum, "wait for reply"=FALSE, "DI Channel Setting"={"DI Channel"=[]}} ("REQ Initialize DI Argument"), "Boolean"=w116, "Wait Notifier"=w114, "wait for reply"=w113, "DI Channel Setting"=w112) -> (w117:T12)
            n180 = call-poly <vilib>:"Delacor_lib_QMH_Enqueue Message (poly).vi"("Message Data"=w117, "Message"="REQ Initialize DI", "Message Queue in"=w120) -> ("error out"=w115:errorcluster)  [unwired: 7 in, 1 out]
          }
          event User Event {
            # "Another Module called the \"REQ Initialize DO\" API Method."
            n181 = event-data() -> ("Boolean"=w125:bool, "Wait Notifier"=w123:refnum<notifier>, "wait for reply"=w122:bool, "DO Channel Setting"=w121:T5)  [unwired: 1 in]
            n182 = Bundle(cluster=T13 {"Boolean"=FALSE, "Wait Notifier"=refnum, "wait for reply"=FALSE, "DO Channel Setting"={"DO Channel"=[]}} ("REQ Initialize DO Argument"), "Boolean"=w125, "Wait Notifier"=w123, "wait for reply"=w122, "DO Channel Setting"=w121) -> (w126:T13)
            n183 = call-poly <vilib>:"Delacor_lib_QMH_Enqueue Message (poly).vi"("Message Data"=w126, "Message"="REQ Initialize DO", "Message Queue in"=w129) -> ("error out"=w124:errorcluster)  [unwired: 7 in, 1 out]
          }
          event User Event {
            # "Another Module called the \"REQ Write DO\" API Method."
            n184 = event-data() -> ("DO Value"=w131:bool[])  [unwired: 1 in]
            n185 = Bundle(cluster=T14 {"DO Value"=[]} ("REQ Write DO Argument"), "DO Value"=w131) -> (w132:T14)
            n186 = call-poly <vilib>:"Delacor_lib_QMH_Enqueue Message (poly).vi"("Message Data"=w132, "Message"="REQ Write DO", "Message Queue in"=w135) -> ("error out"=w130:errorcluster)  [unwired: 7 in, 1 out]
          }
          event User Event {
            # "Another Module called the \"REQ Acquire AI\" API Method."
            n187 = event-data() -> ("Acquire AI"=w137:bool)  [unwired: 1 in]
            n188 = Bundle(cluster=T15 {"Acquire AI"=FALSE} ("REQ Acquire AI Argument"), "Acquire AI"=w137) -> (w138:T15)
            n189 = call-poly <vilib>:"Delacor_lib_QMH_Enqueue Message (poly).vi"("Message Data"=w138, "Message"="REQ Acquire AI", "Message Queue in"=w141) -> ("error out"=w136:errorcluster)  [unwired: 7 in, 1 out]
          }
          event User Event {
            # "Another Module called the \"REQ Close Ref\" API Method."
            n190 = event-data() -> ("Boolean"=w143:bool)  [unwired: 1 in]
            n191 = Bundle(cluster=T16 {"Boolean"=FALSE} ("REQ Close Ref Argument"), "Boolean"=w143) -> (w144:T16)
            n192 = call-poly <vilib>:"Delacor_lib_QMH_Enqueue Message (poly).vi"("Message Data"=w144, "Message"="REQ Close Ref", "Message Queue in"=w147) -> ("error out"=w142:errorcluster)  [unwired: 7 in, 1 out]
          }
          event User Event {
            # "Another Module called the \"REQ Write AO\" API Method."
            n193 = event-data() -> ("Value"=w148:dbl[])  [unwired: 1 in]
            n194 = Bundle(cluster=T17 {"Value"=[]} ("REQ Write AO Argument"), "Value"=w148) -> (w150:T17)
            n195 = call-poly <vilib>:"Delacor_lib_QMH_Enqueue Message (poly).vi"("Message Data"=w150, "Message"="REQ Write AO", "Message Queue in"=w153) -> ("error out"=w149:errorcluster)  [unwired: 7 in, 1 out]
          }
          event User Event {
            # "Another Module called the \"REQ Update Sample Rate\" API Method."
            n196 = event-data() -> ("Timing Parameter"=w155:T3)  [unwired: 1 in]
            n197 = Bundle(cluster=T18 {"Timing Parameter"={"rate"=1000.0, "samples per channel"=1000, "sample mode"=10123}} ("REQ Update Sample Rate Argument"), "Timing Parameter"=w155) -> (w156:T18)
            n198 = call-poly <vilib>:"Delacor_lib_QMH_Enqueue Message (poly).vi"("Message Data"=w156, "Message"="REQ Update Sample Rate", "Message Queue in"=w159) -> ("error out"=w154:errorcluster)  [unwired: 7 in, 1 out]
          }
          event User Event {
            # "Another Module called the \"REQ Acquire DI\" API Method."
            n199 = event-data() -> ("Acquire DI"=w161:bool)  [unwired: 1 in]
            n200 = Bundle(cluster=T19 {"Acquire DI"=FALSE} ("REQ Acquire DI Argument"), "Acquire DI"=w161) -> (w162:T19)
            n201 = call-poly <vilib>:"Delacor_lib_QMH_Enqueue Message (poly).vi"("Message Data"=w162, "Message"="REQ Acquire DI", "Message Queue in"=w165) -> ("error out"=w160:errorcluster)  [unwired: 7 in, 1 out]
          }
        }
        n202 = call-dynamic "Delacor_lib_QMH_Error Handler - Event Handling Loop.vi"("error in"=w45, "Message Queue in"=w39) -> ("dup error in"=w44:errorcluster)  [unwired: 8 in, 1 out]
      }
    }
    frame Error {
      # "Synchronize Caller Events.vi will inform Start Module.vi that the module has launched and will let the code calling Start Module.vi register for broadcasts and would permit the caller receive the broadcast that an error occurred at launch time."
      n203 = call-dynamic "Delacor_lib_QMH_Release Message Queue.vi"("error in"=w453, "Message Queue"=w451) -> ("error out"=w452:errorcluster)  [unwired: 9 in]
      n204 = call "Synchronize Caller Events.vi"("Singleton Module Admin in"=w454) -> ("error out"=w459:errorcluster)  [unwired: 9 in, 1 out]
      n205 = call "Module Name--constant.vi"() -> ("Module Name"=w457:string)  [unwired: 11 in]
      n206 = Format Into String(format string="An error occurred during initialization. %s is no longer running.", w457) -> (resulting string=w455:string)  [unwired: 2 in, 1 out]
      n207 = Merge Errors(w452, w459) -> (w460:errorcluster)
      n208 = call "Error Reported.vi"("Additional Information"=w455, "Error"=w460) -> ()  [unwired: 9 in, 1 out]
    }
  }
  n209 = while {
    shift-right: [w468] -> _
    shift-left: -1 -> [w469]
    tunnel: [w467] -> w9
    tunnel: w11 -> [w465]
    tunnel: w10 -> [w464]
    shift-right: [w462] -> _
    shift-left: w1 -> [w463]
    tunnel: "DAQ Type" -> [w461]
    stop <- w466 stop-if-true
    # "Acquire AI"
    n210 = event shown="[0] Timeout" {
      selector: w465 -> [_ _ _]
      dyn-events: _ -> [_ _ _]
      timeout: w469 -> [w475 _ _]
      tunnel: [w475 w497 _] -> w468
      tunnel: w464 -> [w474 w496 w500]
      tunnel: [w473 w496 w500] -> w467
      tunnel: [_ _ w501] -> w466
      tunnel: w463 -> [w472 w494 _]
      tunnel: [w471 w493 _] -> w462
      tunnel: w461 -> [w470 _ _]
      event Timeout {
        n211 = event-data() -> ()  [unwired: 1 in, 1 out]
        n212 = case shown="No Error" w474 {
          selector: w474 -> [w483 w491]
          tunnel: [w479 w490] -> w473
          tunnel: w472 -> [w481 w489]
          tunnel: [w477 w487] -> w471
          tunnel: w470 -> [_ w485]
          frame No Error {
            n213 = Unbundle By Name(w481) -> ("Abstract.lvclass"=w482:refnum<class "Abstract.lvclass">)
            n214 = call-dynamic "Acquire AI.vi"("error in (no error)"=w483, "Abstract in"=w482) -> ("error out"=w480:errorcluster, "Waveform Graph"=w478:dbl[][], "Abstract out"=w476:refnum<class "Abstract.lvclass">)  [unwired: 7 in]
            "AI Data" <- w478
            n215 = Bundle By Name(cluster=w481, "Abstract.lvclass"=w476) -> (w477:T1)
            n216 = call "REQ Broad AI.vi"("error in"=w480, "AI Data"=w478) -> ("error out"=w479:errorcluster)  [unwired: 9 in]
          }
          frame Error {
            n217 = Unbundle By Name(w489) -> ("Abstract.lvclass"=w488:refnum<class "Abstract.lvclass">)
            n218 = global read "Support Global.vi" "AI Setting"() -> (w484:T2)
            n219 = call-dynamic "Initialize AI.vi"("error in (no error)"=w491, "AI Setting"=w484, "DAQ Type"=w485, "Abstract in"=w488) -> ("error out"=w490:errorcluster, "Abstract out"=w486:refnum<class "Abstract.lvclass">)  [unwired: 6 in]
            n220 = Bundle By Name(cluster=w489, "Abstract.lvclass"=w486) -> (w487:T1)
          }
        }
      }
      event "Acquire AI": Value Change {
        n221 = event-data() -> ("NewVal"=w495:bool)  [unwired: 1 in]
        n222 = global read "Support Global.vi" "Abstract.lvclass"() -> (w492:refnum<class "Abstract.lvclass">)
        n223 = Bundle By Name(cluster=w494, "Abstract.lvclass"=w492) -> (w493:T1)
        n224 = Select(t=0, s=w495, f=-1) -> (s? t:f=w497:i32)
      }
      event User Event {
        n225 = event-data() -> ("Wait for Module to stop?"=w501:bool)  [unwired: 1 in]
      }
    }
  }
  n226 = while {
    shift-right: [w509] -> _
    shift-left: -1 -> [w510]
    tunnel: [w508] -> w2
    tunnel: w5 -> [w506]
    tunnel: w4 -> [w505]
    shift-right: [w503] -> _
    shift-left: w1 -> [w504]
    tunnel: "DAQ Type" -> [w502]
    stop <- w507 stop-if-true
    # "Acquire DI"
    n227 = event shown="[0] Timeout" {
      selector: w506 -> [_ _ _]
      dyn-events: _ -> [_ _ _]
      timeout: w510 -> [w516 _ _]
      tunnel: [w516 w538 _] -> w509
      tunnel: w505 -> [w515 w537 w541]
      tunnel: [w514 w537 w541] -> w508
      tunnel: [_ _ w542] -> w507
      tunnel: w504 -> [w513 w535 _]
      tunnel: [w512 w534 _] -> w503
      tunnel: w502 -> [w511 _ _]
      event Timeout {
        n228 = event-data() -> ()  [unwired: 1 in, 1 out]
        n229 = case shown="No Error" w515 {
          selector: w515 -> [w524 w532]
          tunnel: [w518 w531] -> w514
          tunnel: w513 -> [w522 w530]
          tunnel: [w521 w528] -> w512
          tunnel: w511 -> [_ w526]
          frame No Error {
            n230 = Unbundle By Name(w522) -> ("Abstract.lvclass"=w523:refnum<class "Abstract.lvclass">)
            n231 = call-dynamic "Acquire DI.vi"("error in (no error)"=w524, "Abstract in"=w523) -> ("error out"=w519:errorcluster, "Acquire DI"=w517:bool[], "Abstract out"=w520:refnum<class "Abstract.lvclass">)  [unwired: 7 in]
            n232 = Bundle By Name(cluster=w522, "Abstract.lvclass"=w520) -> (w521:T1)
            n233 = call "REQ Broadcast DI.vi"("error in"=w519, "DI"=w517) -> ("error out"=w518:errorcluster)  [unwired: 9 in]
          }
          frame Error {
            n234 = Unbundle By Name(w530) -> ("Abstract.lvclass"=w529:refnum<class "Abstract.lvclass">)
            n235 = global read "Support Global.vi" "DI  Setting"() -> (w525:T4)
            n236 = call-dynamic "Initialize DI.vi"("error in (no error)"=w532, "DI Channel Setting"=w525, "DAQ Type"=w526, "Abstract in"=w529) -> ("error out"=w531:errorcluster, "Abstract out"=w527:refnum<class "Abstract.lvclass">)  [unwired: 6 in]
            n237 = Bundle By Name(cluster=w530, "Abstract.lvclass"=w527) -> (w528:T1)
          }
        }
      }
      event "Acquire DI": Value Change {
        n238 = event-data() -> ("NewVal"=w536:bool)  [unwired: 1 in]
        n239 = global read "Support Global.vi" "Abstract.lvclass"() -> (w533:refnum<class "Abstract.lvclass">)
        n240 = Bundle By Name(cluster=w535, "Abstract.lvclass"=w533) -> (w534:T1)
        n241 = Select(t=0, s=w536, f=-1) -> (s? t:f=w538:i32)
      }
      event User Event {
        n242 = event-data() -> ("Wait for Module to stop?"=w542:bool)  [unwired: 1 in]
      }
    }
  }
  n243 = Merge Errors(w26, w28, w9, w2) -> (w25:errorcluster)
  n244 = call "Close Module.vi"("error in (no error)"=w25, "Module Admin in"=w23) -> ("error out"=w27:errorcluster, "External Launch"=w19:bool, "Module Admin out"=w20:refnum<class "Delacor_lib_QMH_Module Admin.lvclass">)  [unwired: 7 in]
  n245 = Unregister For Events(event registration refnum=w22, error in=w27) -> (error out=w24:errorcluster)
  "error out" <- w24
  n246 = case "External Launch?" shown="True" w19 {
    tunnel: w24 -> [_ w543]
    frame False {
    }
    frame True {
      n247 = case shown="No Error" w543 {
        frame No Error {
          n248 = invoke class="VI" method="FP.Close"() -> ()  [unwired: 3 in, 3 out]
        }
        frame Error {
          n249 = invoke class="VI" method="FP.Open"("Activate"=TRUE ("Activate?")) -> ()  [unwired: 4 in, 5 out]
        }
      }
    }
  }
  n250 = local write "Module Admin"(w20) -> ()
